vi "ChipSlotSelect.vi"() -> ()   [LabVIEW 2014]
uses:
  g_CipHolderConstants.vi
  g_ChipData.vi
panel:
  in  "OK":bool
  in  "Modify":bool
  in  "Unselect":bool
  in  "Select":bool
  in  "Occupied":bool[][](array[boolean])
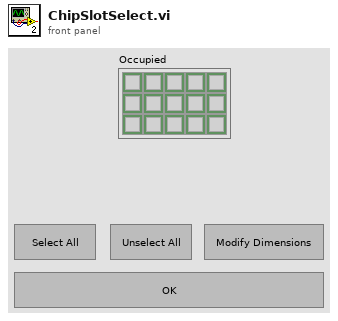
[diagram p1: front panel]
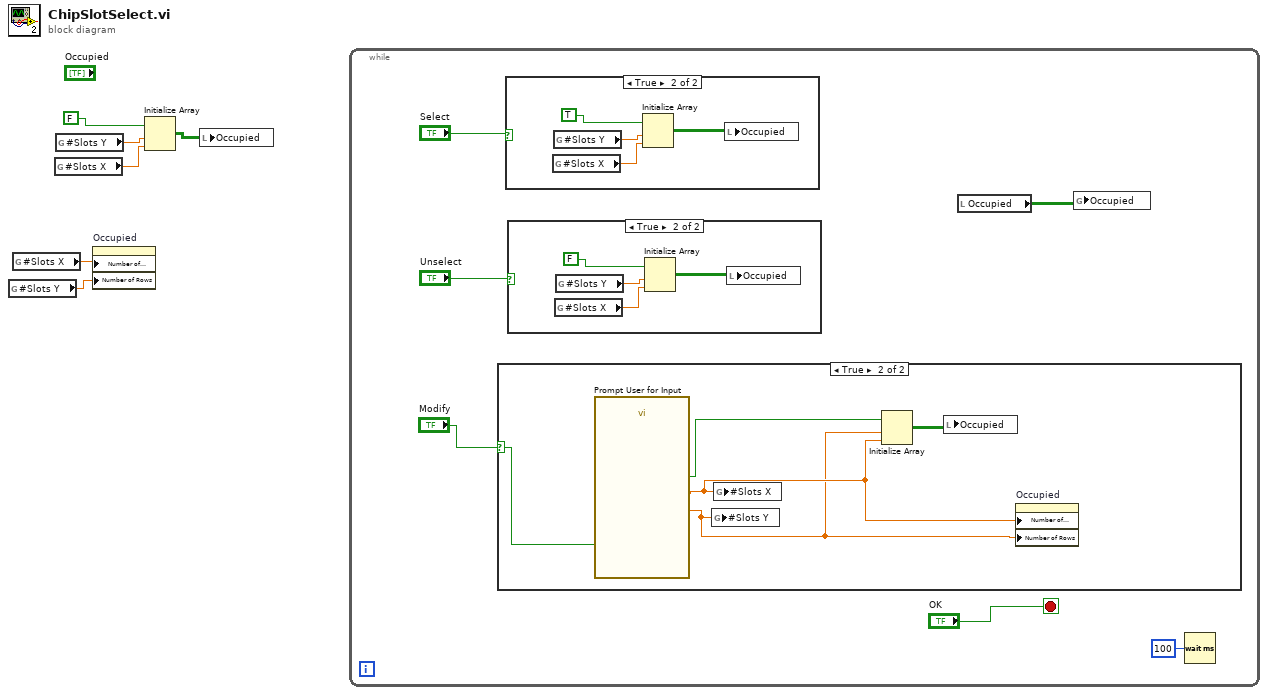
[diagram p0: block diagram]
diagram:
  n1 = global read "g_CipHolderConstants.vi" "#Slots Y"() -> (w2:dbl)
  n2 = global read "g_CipHolderConstants.vi" "#Slots X"() -> (w1:dbl)
  n3 = global read "g_CipHolderConstants.vi" "#Slots X"() -> (w5:dbl)
  n4 = global read "g_CipHolderConstants.vi" "#Slots Y"() -> (w6:dbl)
  n5 = property on="Occupied" class="Arr (strict)"("Number of Columns"=w1, "Number of Rows"=w2) -> ()  [unwired: 2 in, 2 out]
  n6 = Initialize Array(FALSE, w6, w5) -> (w3:bool[][])
  n7 = local write "Occupied"(w3) -> ()
  n8 = while {
    stop <- "OK" stop-if-true
    n9 = case shown="True" "Modify" {
      selector: "Modify" -> [_ w17]
      frame False {
      }
      frame True {
        n10 = call "Prompt User for Input"("Enable"=w17) -> ("# Chipslots along Y axis"=w13:dbl, "# Chipslots along X axis"=w14:dbl, "OK"=w16:bool)  [unwired: 15 in, 1 out]
        n11 = global write "g_CipHolderConstants.vi" "#Slots Y"(w13) -> ()
        n12 = global write "g_CipHolderConstants.vi" "#Slots X"(w14) -> ()
        n13 = Initialize Array(w16, w13, w14) -> (w15:bool[][])
        n14 = local write "Occupied"(w15) -> ()
        n15 = property on="Occupied" class="Arr (strict)"("Number of Columns"=w14, "Number of Rows"=w13) -> ()  [unwired: 2 in, 2 out]
      }
    }
    n16 = case shown="True" "Select" {
      frame False {
      }
      frame True {
        n17 = global read "g_CipHolderConstants.vi" "#Slots X"() -> (w23:dbl)
        n18 = global read "g_CipHolderConstants.vi" "#Slots Y"() -> (w22:dbl)
        n19 = Initialize Array(TRUE, w22, w23) -> (w25:bool[][])
        n20 = local write "Occupied"(w25) -> ()
      }
    }
    n21 = case shown="True" "Unselect" {
      frame False {
      }
      frame True {
        n22 = global read "g_CipHolderConstants.vi" "#Slots X"() -> (w19:dbl)
        n23 = global read "g_CipHolderConstants.vi" "#Slots Y"() -> (w18:dbl)
        n24 = Initialize Array(FALSE, w18, w19) -> (w21:bool[][])
        n25 = local write "Occupied"(w21) -> ()
      }
    }
    n26 = local read "Occupied"() -> (w9:bool[][])
    n27 = global write "g_ChipData.vi" "Occupied"(w9) -> ()
    n28 = Wait (ms)(milliseconds to wait=u32 100) -> ()  [unwired: 1 out]
  }
